vi "color_normalization_cluster.vi"(11 "Color tables array":T1[](array[typedef])=[enum."Grayscale"]) -> (3 "Normalization cluster":cluster{"[0]":dbl, "[1]":dbl, "[2]":dbl})   [LabVIEW 2011, in "Fiberscope_library.lvlib"]
uses:
  Fiberscope_library.lvlib
  typedefs/color_palette_enum.ctl
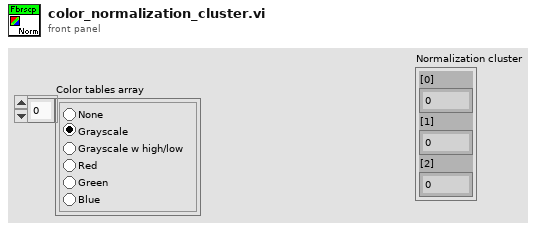
[diagram p1: front panel]
types:
  T1 = typedef "Fiberscope_library.lvlib/color_palette_enum.ctl" = enum32{"None", "Grayscale", "Grayscale w high/low", "Red", "Green", "Blue"}
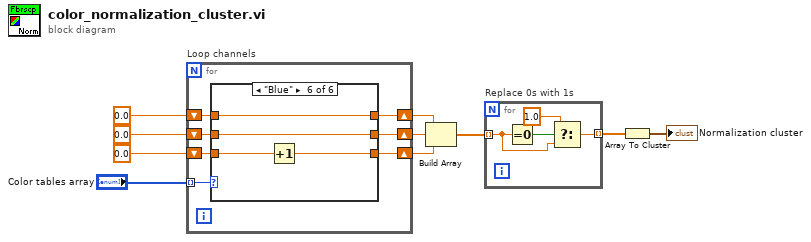
[diagram p0: block diagram]
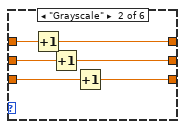
[diagram p3: hidden frame]
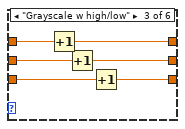
[diagram p4: hidden frame]
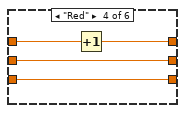
[diagram p5: hidden frame]
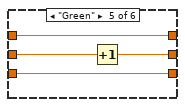
[diagram p6: hidden frame]
diagram:
  n1 = for "Loop channels" {
    tunnel: "Color tables array" -> [w14] mode=indexing
    shift-right: [w13] -> w3
    shift-left: 0.0 ("element") -> [w17]
    shift-right: [w12] -> w2
    shift-left: 0.0 ("element") -> [w16]
    shift-right: [w11] -> w1
    shift-left: 0.0 ("element") -> [w15]
    n2 = case shown="\"Blue\"" w14 {
      tunnel: w17 -> [w20 w26 w32 w36 w38 w41]
      tunnel: w16 -> [w19 w25 w31 w34 w40 w42]
      tunnel: w15 -> [w18 w24 w30 w33 w37 w44]
      tunnel: [w20 w23 w29 w35 w38 w41] -> w13
      tunnel: [w19 w22 w28 w34 w39 w42] -> w12
      tunnel: [w18 w21 w27 w33 w37 w43] -> w11
      frame "None", Default {
      }
      frame "Grayscale" {
        n3 = Increment(x=w26) -> (x+1=w23:dbl)
        n4 = Increment(x=w25) -> (x+1=w22:dbl)
        n5 = Increment(x=w24) -> (x+1=w21:dbl)
      }
      frame "Grayscale w high/low" {
        n6 = Increment(x=w32) -> (x+1=w29:dbl)
        n7 = Increment(x=w31) -> (x+1=w28:dbl)
        n8 = Increment(x=w30) -> (x+1=w27:dbl)
      }
      frame "Red" {
        n9 = Increment(x=w36) -> (x+1=w35:dbl)
      }
      frame "Green" {
        n10 = Increment(x=w40) -> (x+1=w39:dbl)
      }
      frame "Blue" {
        n11 = Increment(x=w44) -> (x+1=w43:dbl)
      }
    }
  }
  n12 = Build Array(w3, w2, w1) -> (w8:dbl[])
  n13 = for "Replace 0s with 1s" {
    tunnel: [w46] -> w9 mode=indexing
    tunnel: w8 -> [w45] mode=indexing
    n14 = Equal To 0?(x=w45) -> (x = 0?=w48:bool)
    n15 = Select(t=1.0, s=w48, f=w45) -> (s? t:f=w46:dbl)
  }
  n16 = Array To Cluster(array=w9) -> (cluster=→"Normalization cluster":cluster{"[0]":dbl, "[1]":dbl, "[2]":dbl})
